vi "Attenuator_Control.vi"(3 "错误输入":errorcluster, 4 "位置":T2, 5 "控制电机指令":T1, 6 "电机":T3) -> (0 "error out":errorcluster caption="错误输出", 1 "通信成功？":bool)   [LabVIEW 2018]
panel:
  in  "Position":i32
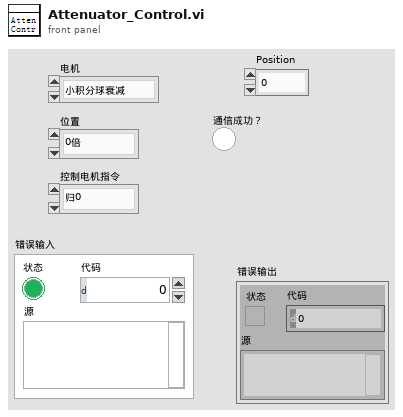
[diagram p1: front panel]
types:
  T1 = typedef "衰减片电机指令枚举器.ctl" = enum16{"归0", "停止", "运动", "轴设置", "通信连接", "读取位置"}
  T2 = typedef "衰减片电机位置枚举器.ctl" = enum16{"0倍", "10倍", "100倍", "1000倍"}
  T3 = typedef "衰减片电机枚举.ctl" = enum16{"小积分球衰减", "偏振仪衰减", "近场相机衰减", "远场相机衰减"}
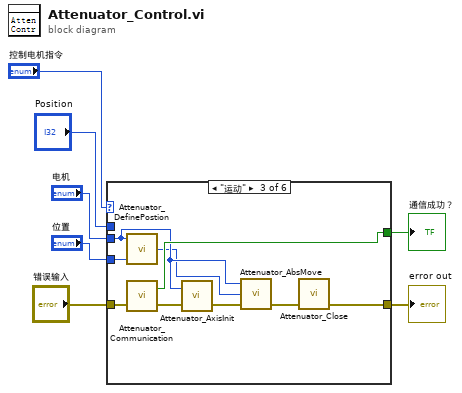
[diagram p0: block diagram]
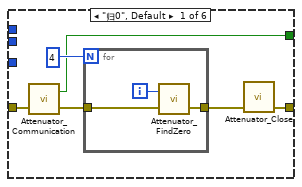
[diagram p2: hidden frame]
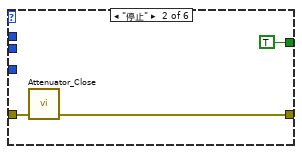
[diagram p3: hidden frame]
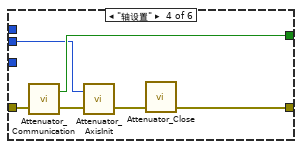
[diagram p4: hidden frame]
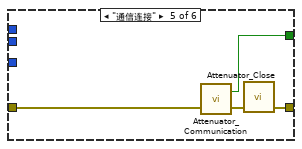
[diagram p5: hidden frame]
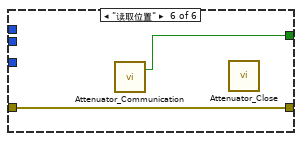
[diagram p6: hidden frame]
diagram:
  n1 = case shown="\"运动\"" "控制电机指令" {
    tunnel: [w11 TRUE ("通信成功？") w28 w33 w37 w39] -> w6
    tunnel: "电机" -> [_ _ w24 w32 _ _]
    tunnel: "Position" -> [_ _ _ _ _ _]
    tunnel: "位置" -> [_ _ w23 _ _ _]
    tunnel: "错误输入" -> [w9 w18 w21 w30 w36 w40]
    tunnel: [w8 w17 w20 w29 w35 w40] -> w1
    frame "归0", Default {
      n2 = call "Attenuator_Communication.vi"("错误输入"=w9) -> ("错误输出"=w12:errorcluster, "通信成功？"=w11:bool)  [unwired: 1 in]
      n3 = for {
        N: 4 -> [_]
        tunnel: w12 -> [w15]
        tunnel: [w14] -> w10
        i -> [w16]
        n4 = call "Attenuator_FindZero.vi"("error in (no error)"=w15, "Axis"=w16) -> ("error out"=w14:errorcluster)  [unwired: 1 in]
      }
      n5 = call "Attenuator_Close.vi"("error in (no error)"=w10) -> ("error out"=w8:errorcluster)  [unwired: 4 in]
    }
    frame "停止" {
      n6 = call "Attenuator_Close.vi"("error in (no error)"=w18) -> ("error out"=w17:errorcluster)  [unwired: 4 in]
    }
    frame "运动" {
      n7 = call "Attenuator_DefinePostion.vi"("位置"=w23, "电机"=w24) -> ("PosOut"=w22:i32)  [unwired: 3 in]
      n8 = call "Attenuator_Communication.vi"("错误输入"=w21) -> ("错误输出"=w27:errorcluster, "通信成功？"=w28:bool)  [unwired: 1 in]
      n9 = call "Attenuator_AxisInit.vi"("error in (no error)"=w27, "Axis"=w24) -> ("error out"=w26:errorcluster)  [unwired: 1 in]
      n10 = call "Attenuator_AbsMove.vi"("error in (no error)"=w26, "Position"=w22, "Axis"=w24) -> ("error out"=w25:errorcluster)  [unwired: 2 in]
      n11 = call "Attenuator_Close.vi"("error in (no error)"=w25) -> ("error out"=w20:errorcluster)  [unwired: 4 in]
    }
    frame "轴设置" {
      n12 = call "Attenuator_Communication.vi"("错误输入"=w30) -> ("错误输出"=w34:errorcluster, "通信成功？"=w33:bool)  [unwired: 1 in]
      n13 = call "Attenuator_AxisInit.vi"("error in (no error)"=w34, "Axis"=w32) -> ("error out"=w31:errorcluster)  [unwired: 1 in]
      n14 = call "Attenuator_Close.vi"("error in (no error)"=w31) -> ("error out"=w29:errorcluster)  [unwired: 4 in]
    }
    frame "通信连接" {
      n15 = call "Attenuator_Communication.vi"("错误输入"=w36) -> ("错误输出"=w38:errorcluster, "通信成功？"=w37:bool)  [unwired: 1 in]
      n16 = call "Attenuator_Close.vi"("error in (no error)"=w38) -> ("error out"=w35:errorcluster)  [unwired: 4 in]
    }
    frame "读取位置" {
      n17 = call "Attenuator_Communication.vi"() -> ("通信成功？"=w39:bool)  [unwired: 2 in, 1 out]
      n18 = call "Attenuator_Close.vi"() -> ()  [unwired: 5 in, 1 out]
    }
  }
  "通信成功？" <- w6
  "error out" <- w1
